vi "Create Bus Log File.vi"(10 "Addon":string, 11 "Project Folder":path) -> (0 "error out":errorcluster, 1 "Continue":bool, 2 "Status":string, 3 "Byte Stream File out":refnum<file>)   [LabVIEW 2019, in "CAN Stream Support Workspace Shared.lvlib"]
uses:
  CAN Stream Support Workspace Shared.lvlib
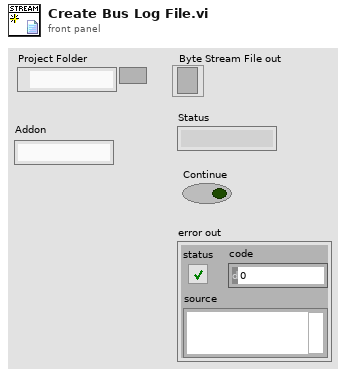
[diagram p1: front panel]
types:
  T1 = enum16{"open", "replace", "create", "open or create", "replace or create", "replace or create with confirmation"}
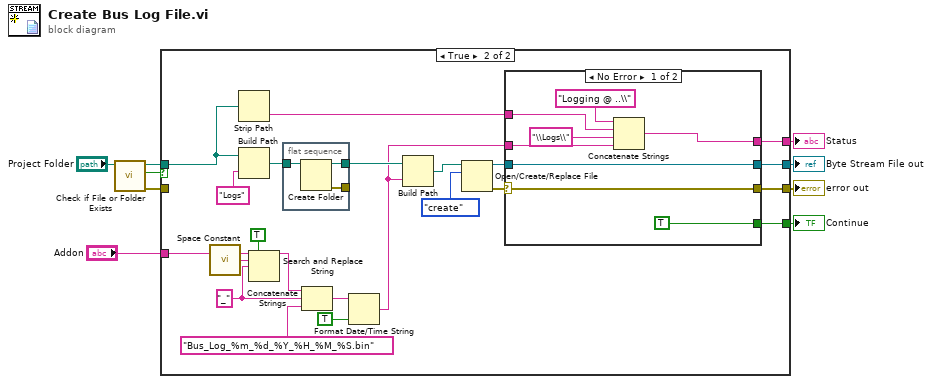
[diagram p0: block diagram]
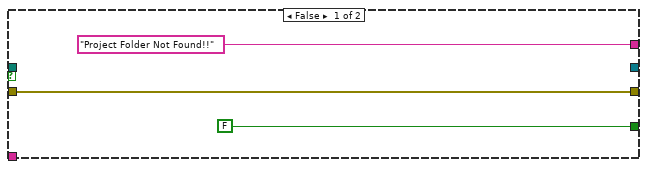
[diagram p2: hidden frame]
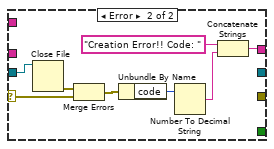
[diagram p3: hidden frame]
diagram:
  n1 = call <vilib>:"Check if File or Folder Exists.vi"("path"="Project Folder") -> ("error out"=w9:errorcluster, "file or folder exists?"=w8:bool, "dup path"=w7:path)  [unwired: 8 in]
  n2 = case shown="True" w8 {
    tunnel: [w11 w33] -> w2
    tunnel: [_ w32] -> w3
    tunnel: [FALSE w30] -> w4
    tunnel: ["Project Folder Not Found!!" w25] -> w5
    tunnel: w7 -> [_ w20]
    tunnel: w9 -> [w11 _]
    tunnel: "Addon" -> [_ w19]
    frame False {
    }
    frame True {
      w15 = "_" ("replace string (\"\")")
      n3 = call <vilib>:"Space Constant.vi"() -> ("String"=w17:string)
      n4 = Strip Path(path=w20) -> (name=w21:string)  [unwired: 1 out]
      n5 = Build Path(base path=w20, name or relative path="Logs") -> (appended path=w23:path)
      n6 = Search and Replace String(replace all?=TRUE ("replace all? (F)"), input string=w19, search string=w17, replace string=w15) -> (result string=w16:string)  [unwired: 4 in, 3 out]
      n7 = flat-sequence {
        tunnel: w23 -> [w37]
        tunnel: [w36] -> _
        tunnel: [w35] -> w27
        frame #0 {
          n8 = Create Folder(path (use dialog)=w37) -> (created path=w35:path, error out=w36:errorcluster)  [unwired: 2 in, 1 out]
        }
      }
      n9 = Concatenate Strings(w16, w15, "Bus_Log_%m_%d_%Y_%H_%M_%S.bin" ("time format string (%c)")) -> (w13:string)
      n10 = Format Date/Time String(time format string (%c)=w13, UTC format=TRUE) -> (date/time string=w22:string)  [unwired: 1 in]
      n11 = Build Path(base path=w27, name or relative path=w22) -> (appended path=w26:path)
      n12 = Open/Create/Replace File(file path (use dialog)=w26, operation (0:open)=T1."create") -> (refnum out=w34:refnum<file>, error out=w31:errorcluster)  [unwired: 4 in, 1 out]
      n13 = case shown="No Error" w31 {
        selector: w31 -> [w44 w51]
        tunnel: w34 -> [w43 w53]
        tunnel: [w44 _] -> w33
        tunnel: [w43 _] -> w32
        tunnel: [TRUE _] -> w30
        tunnel: [w41 w46] -> w25
        tunnel: w22 -> [w38 _]
        tunnel: w21 -> [w40 _]
        frame No Error {
          n14 = Concatenate Strings("Logging @ ..\\" ("string"), w40, "\\Logs\\" ("string"), w38) -> (w41:string)
        }
        frame Error {
          n15 = Close File(refnum=w53) -> (error out=w52:errorcluster)  [unwired: 1 in, 1 out]
          n16 = Merge Errors(w52, w51) -> (w50:errorcluster)
          n17 = Unbundle By Name(w50) -> ("code"=w49:i32)
          n18 = Number To Decimal String(number=w49) -> (decimal integer string=w48:string)  [unwired: 1 in]
          n19 = Concatenate Strings("Creation Error!! Code: ", w48) -> (w46:string)
        }
      }
    }
  }
  "Status" <- w5
  "Continue" <- w4
  "Byte Stream File out" <- w3
  "error out" <- w2
